vi "Main.vi"(11 "Module Admin":refnum<class "Delacor_lib_QMH_Cloneable Module Admin.lvclass">) -> ()   [LabVIEW 2024, in "OtroClon.lvlib"]
doc: "This template is based off of the Queued Message Handler design pattern and the Queued Message Handler project template that ships with LabVIEW.\n\nThe main difference is that the queue is private to this module and communication between modules is performed via Broadcast and Request events.\n\nRequest events are wrapped in public API methods and are handled in the Event Handling Loop (EHL) of this VI. Any module can register for Broadcast events sent by this module. The EHL generates messages based on user interface actions.\n\nThe Message Handling Loop (MHL) processes messages generated by the EHL, or by other messages. The messages are string values, so new messages can be added easily to the Message Cases case structure in the MHL. Each message cluster can also provide an optional value for Message Data, which is a variant that can be converted to whatever message-specific data is required.\n_____\nBased on DQMH Dev Tools: Project Template 7.1.0.1503."
uses:
  OtroClon.lvlib
  <vilib>/Delacor/Delacor QMH/Libraries/Cloneable Module Admin_class/Delacor_lib_QMH_Cloneable Module Admin.lvclass
  C:/Program Files (x86)/National Instruments/LabVIEW 2024/vi.lib/Delacor/Delacor QMH/Libraries/Module Admin_class/Delacor_lib_QMH_Module Admin.lvclass
  Module Data--cluster.ctl
  Do Something Argument--cluster.ctl
  <vilib>/Delacor/Delacor QMH/Libraries/Cloneable Module Admin_class/Delacor_lib_QMH_Cloneable Module Admin.lvclass/Delacor_lib_QMH_Cloneable Module Admin.ctl
  <vilib>/Delacor/Delacor QMH/Libraries/Message Queue_class/Delacor_lib_QMH_Message Queue.lvclass/Delacor_lib_QMH_Message Queue.ctl
  Do Something Else Argument--cluster.ctl
  Do Something Else and Wait for Reply Argument--cluster.ctl
  Do Something Else and Wait (Reply Payload)--cluster.ctl
  Stop Argument--cluster.ctl
  <vilib>/Delacor/Delacor QMH/Libraries/Module Admin_class/Delacor_lib_QMH_Module Admin.lvclass/Delacor_lib_QMH_Module Admin.ctl
  Evento Demo Copia Argument--cluster.ctl
  Set Signal Type Argument--cluster.ctl
  <vilib>/Utility/miscctls.llb/LVPointTypeDef.ctl
  <vilib>/Delacor/Delacor QMH/Libraries/Message Queue_class/Delacor_lib_QMH_Enqueue Message (Single).vi
  <vilib>/Delacor/Delacor QMH/Libraries/Cloneable Module Admin_class/Delacor_lib_QMH_Get Module ID.vi
  <vilib>/Delacor/Delacor QMH/Libraries/Module Admin_class/Delacor_lib_QMH_Get External Launch.vi
  <vilib>/Delacor/Delacor QMH/Libraries/Message Queue_class/Delacor_lib_QMH_Message Queue.lvclass
panel:
  out "error out":errorcluster
  out "X":dbl
  out "Status":string
  in  "Simulate EHL Error":bool
  in  "Simulate MHL Error":bool
  in  "Do Something Else <Replace Me>":bool
  in  "Do Something <Replace Me>":bool
  # "These controls have associated \"Value Changed\" events configured in the Event Structure on the diagram.\n\nReplace them (and reconfigure the Event Structure) with the controls you need for your application. \n\nOther processes communicate with this Module via its Public API (wrappers for its Request Events).\n\nThis Module communicates with other processes via its Broadcast Events.\nAny process that wants to receive these messages can register for this module's Broadcast events."
  # "This template is for the DQMH framework. See the block diagram for more information on how to use this template."
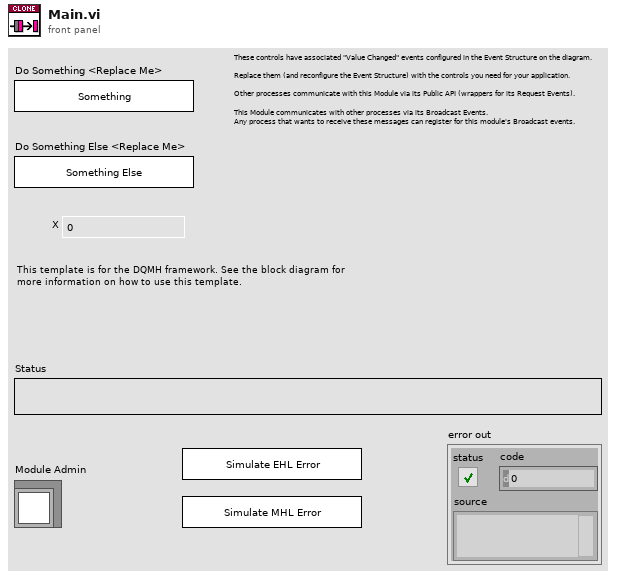
[diagram p1: front panel]
types:
  T1 = typedef "OtroClon.lvlib/Request Events--cluster.ctl" = cluster{"Stop Module":refnum<user-event>, "Do Something":refnum<user-event>, "Do Something Else":refnum<user-event>, "Do Something Else and Wait for Reply":refnum<user-event>, "Show Panel":refnum<user-event>, "Hide Panel":refnum<user-event>, "Show Diagram":refnum<user-event>, "Get Module Execution Status":refnum<user-event>, "Evento Demo Copia":refnum<user-event>, "Set Signal Type":refnum<user-event>}
  T2 = typedef "OtroClon.lvlib/Module Data--cluster.ctl" = cluster{"Status":string, "signal type":enum16{"Sine Wave", "Triangle Wave", "Square Wave", "Sawtooth Wave"}}
  T3 = typedef "OtroClon.lvlib/Do Something Argument--cluster.ctl" = cluster{"Module ID":i32, "Do Something Msg":string}
  T4 = typedef "OtroClon.lvlib/Do Something Else Argument--cluster.ctl" = cluster{"Module ID":i32, "Do Something Else Msg":string, "X":dbl}
  T5 = typedef "OtroClon.lvlib/Do Something Else and Wait for Reply Argument--cluster.ctl" = cluster{"Module ID":i32, "Do Something Else Msg":string, "X":dbl, "Wait Notifier":refnum<notifier>, "wait for reply":bool}
  T6 = enum32{"invalid lock state", "Not Locked", "Locked (No Password)", "Password-protected"}
  T7 = typedef "OtroClon.lvlib/Stop Argument--cluster.ctl" = cluster{"Module ID":i32, "Origin":string, "Exit via Stop Module Req?":bool, "Wait for Module to stop?":bool}
  T8 = typedef "OtroClon.lvlib/Evento Demo Copia Argument--cluster.ctl" = cluster{"Module ID":i32, "Numeric":dbl}
  T9 = typedef "OtroClon.lvlib/Set Signal Type Argument--cluster.ctl" = cluster{"Module ID":i32, "signal type":enum16{"Sine Wave", "Triangle Wave", "Square Wave", "Sawtooth Wave"}}
  T10 = typedef "LVPointTypeDef.ctl" = cluster{"Horizontal":i16, "Vertical":i16}
  T11 = enum32{"Invalid", "Standard", "Closed", "Hidden", "Minimized", "Maximized"}
  T12 = typedef "OtroClon.lvlib/Do Something Else and Wait (Reply Payload)--cluster.ctl" = cluster{"Value":dbl, "error":errorcluster, "Module ID":i32}
  T13 = enum16{"Sine Wave", "Triangle Wave", "Square Wave", "Sawtooth Wave"}
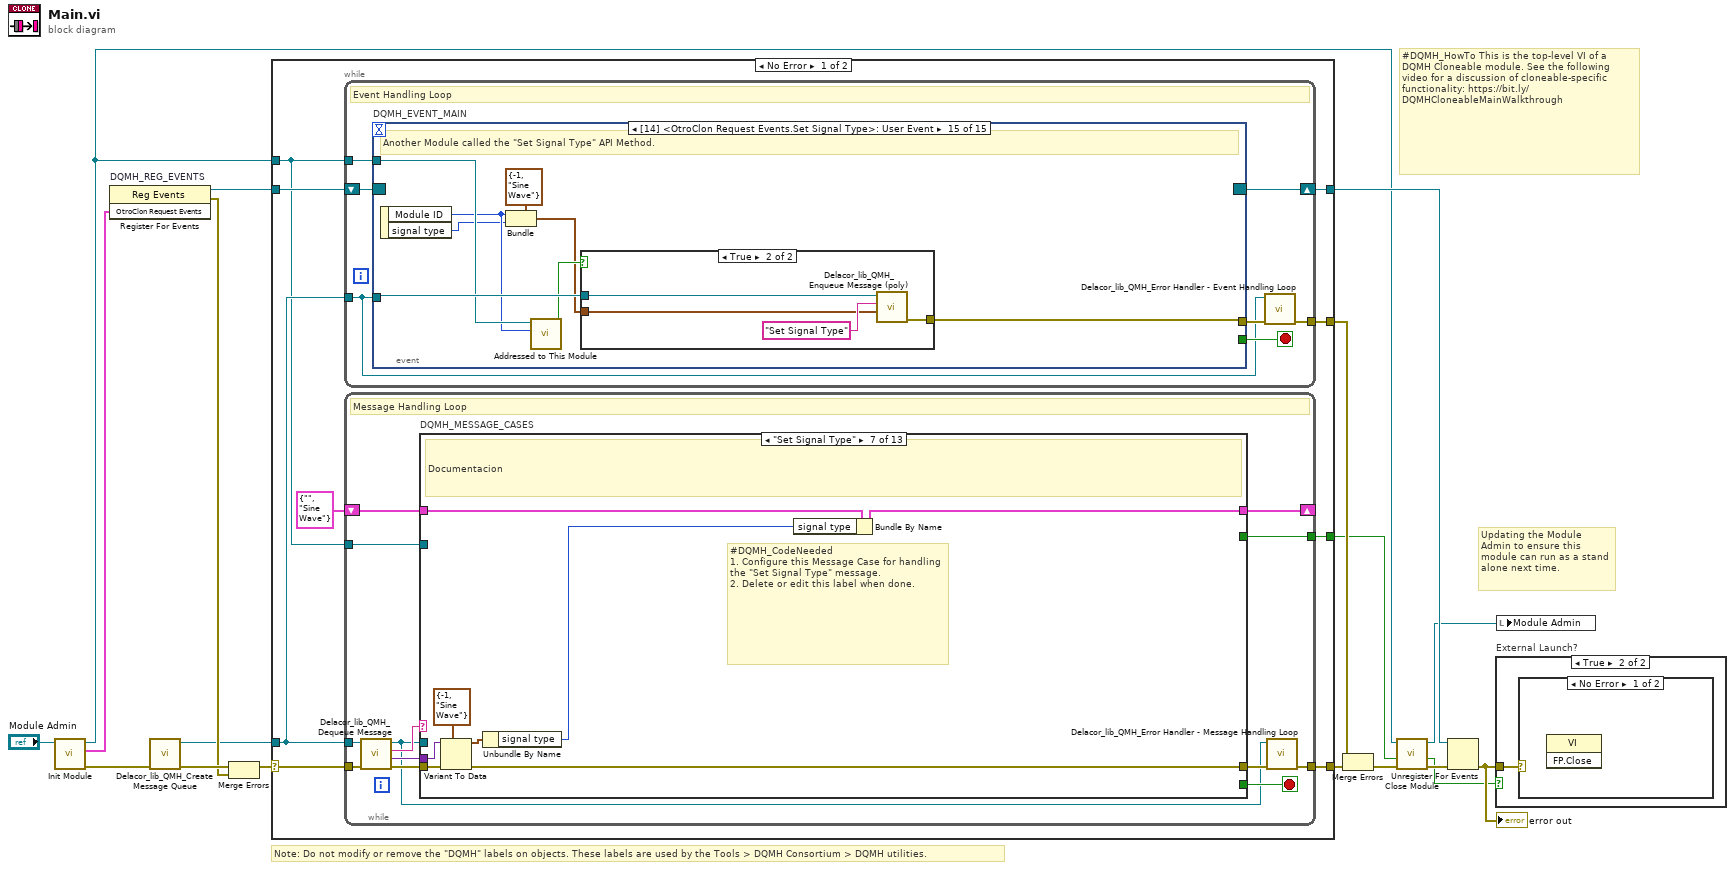
[diagram p0: block diagram]
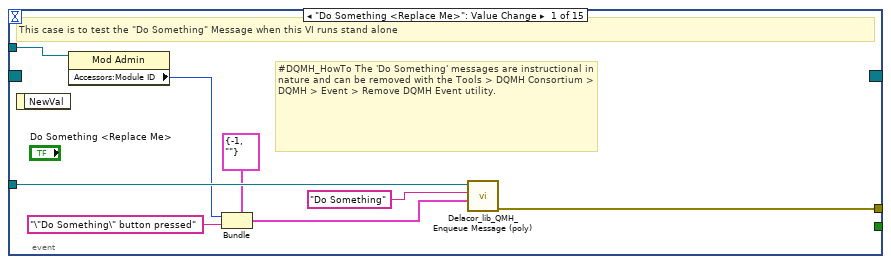
[diagram p2: hidden frame]
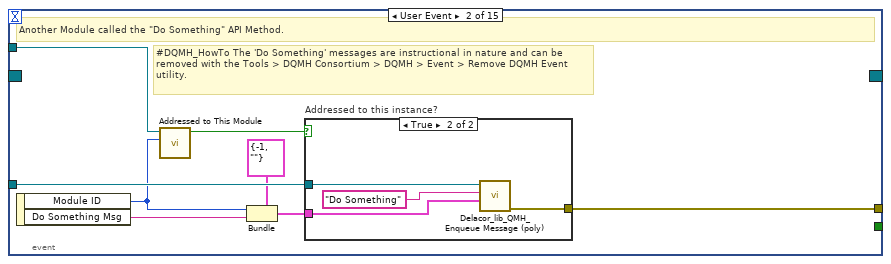
[diagram p3: hidden frame]
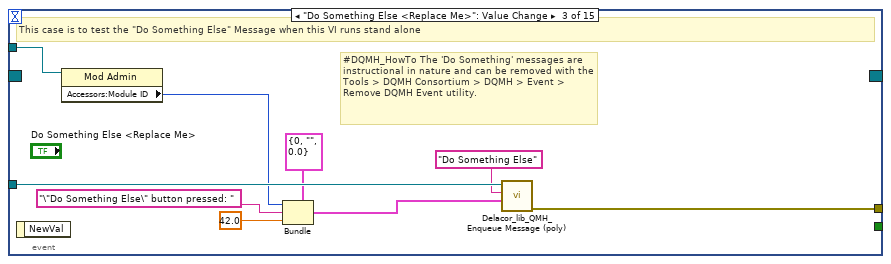
[diagram p5: hidden frame]
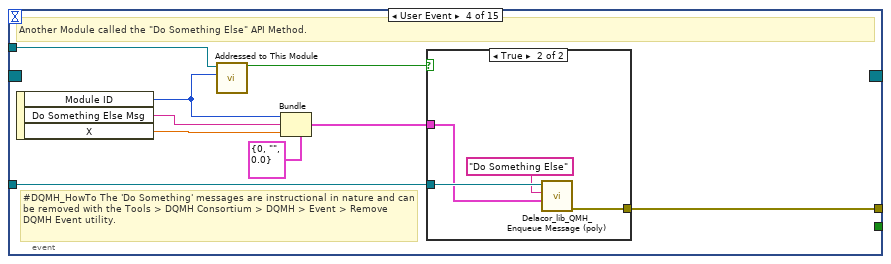
[diagram p6: hidden frame]
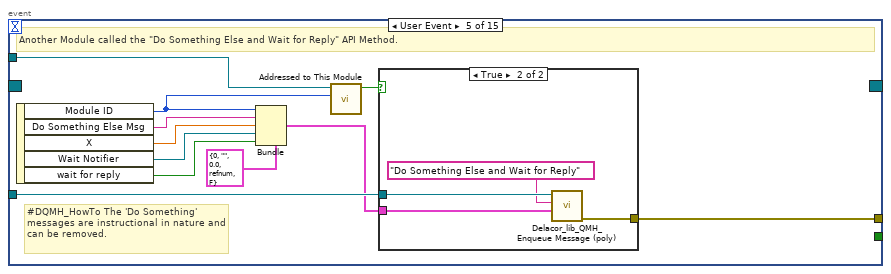
[diagram p8: hidden frame]
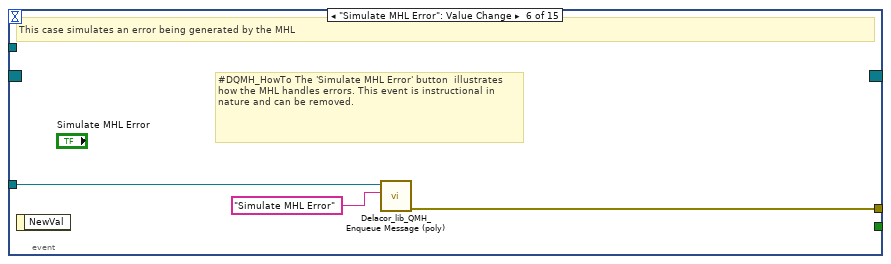
[diagram p10: hidden frame]
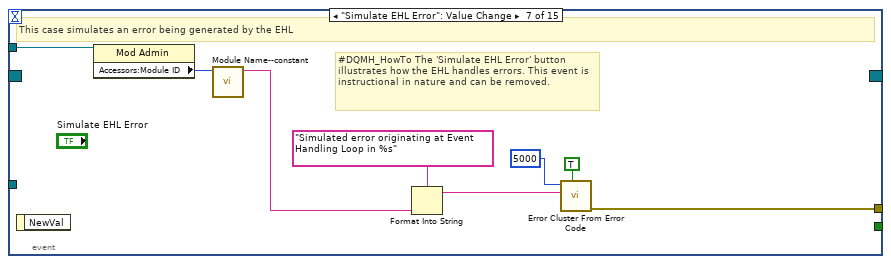
[diagram p11: hidden frame]
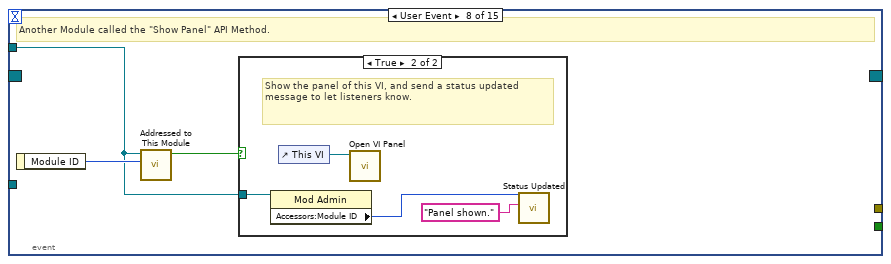
[diagram p12: hidden frame]
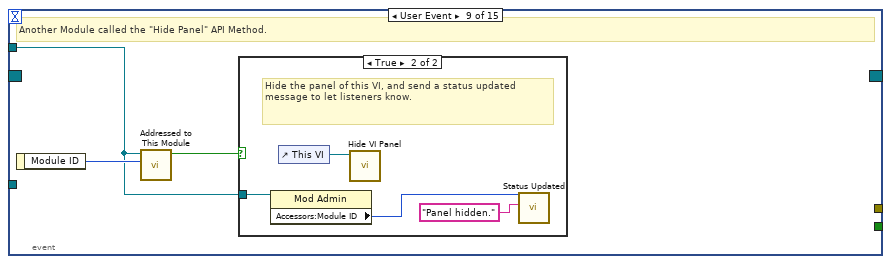
[diagram p14: hidden frame]
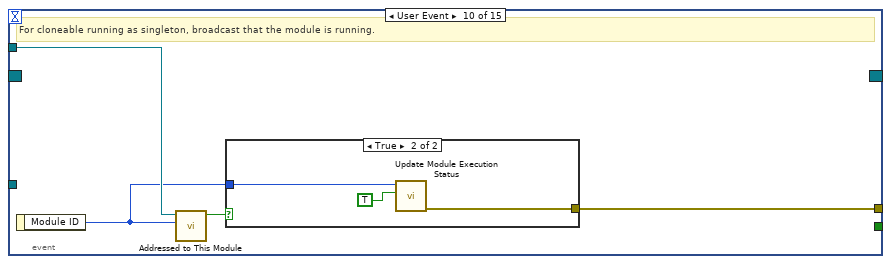
[diagram p16: hidden frame]
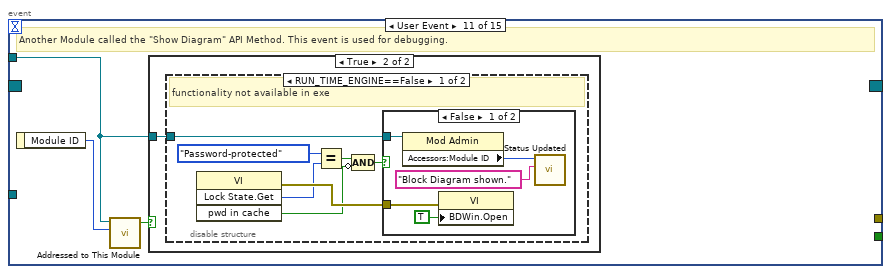
[diagram p18: hidden frame]
diagram:
  # "#DQMH_HowTo This is the top-level VI of a DQMH Cloneable module. See the following video for a discussion of cloneable-specific functionality: https://bit.ly/DQMHCloneableMainWalkthrough"
  # "Note: Do not modify or remove the \"DQMH\" labels on objects. These labels are used by the Tools > DQMH Consortium > DQMH utilities."
  # "Updating the Module Admin to ensure this module can run as a stand alone next time."
  n1 = call "Init Module.vi"("Cloneable Module Admin in"="Module Admin") -> ("error out"=w15:errorcluster, "OtroClon Request Events"=w7:T1, "Cloneable Module Admin out"=w4:refnum<class "Delacor_lib_QMH_Cloneable Module Admin.lvclass">)  [unwired: 8 in]
  n2 = register-events "DQMH_REG_EVENTS"(w7) -> (reference out=w8:refnum<event-registration>, error out=w10:errorcluster)  [unwired: 2 in]
  n3 = call <vilib>:"Delacor_lib_QMH_Create Message Queue.vi"("error in"=w15) -> ("error out"=w12:errorcluster, "Message Queue"=w6:refnum<class "Delacor_lib_QMH_Message Queue.lvclass">)  [unwired: 9 in]
  n4 = Merge Errors(w12, w10) -> (w11:errorcluster)
  n5 = case shown="No Error" w11 {
    selector: w11 -> [w25 w374]
    tunnel: [w27 w373] -> w16
    tunnel: [w24 w372] -> w9
    tunnel: w8 -> [w22 w372]
    tunnel: w6 -> [w21 w365]
    tunnel: [w26 _] -> w17
    tunnel: w4 -> [w20 w368]
    tunnel: [w19 _] -> w2
    frame No Error {
      n6 = while {
        tunnel: w21 -> [w28]
        shift-right: [w31] -> w24
        shift-left: w22 -> [w32]
        tunnel: [w33] -> w26
        tunnel: w20 -> [w29]
        stop <- w30 stop-if-true
        # "Event Handling Loop"
        n7 = event "DQMH_EVENT_MAIN" shown="[14] <OtroClon Request Events.Set Signal Type>: User Event" {
          selector: w32 -> [_ _ _ _ _ _ _ _ _ _ _ _ _ _ _]
          dyn-events: [_ _ _ _ _ _ _ _ _ _ _ _ _ _ _] -> w31
          timeout: _ -> [_ _ _ _ _ _ _ _ _ _ _ _ _ _ _]
          tunnel: [_ _ _ _ _ _ _ _ _ _ _ w143 _ _ _] -> w30
          tunnel: w28 -> [w41 w49 w62 w71 w86 w93 _ _ _ _ _ w146 w163 w183 w195]
          tunnel: [w42 w50 w63 w72 w87 w94 w102 _ _ w120 _ w147 w166 w176 w188] -> w34
          tunnel: w29 -> [w37 w47 w56 w69 w84 _ w101 w103 w110 w118 w124 w145 w164 w181 w193]
          event "Do Something <Replace Me>": Value Change {
            # "#DQMH_HowTo The 'Do Something' messages are instructional in nature and can be removed with the Tools > DQMH Consortium > DQMH > Event > Remove DQMH Event utility."
            # "This case is to test the \"Do Something\" Message when this VI runs stand alone"
            n8 = event-data() -> ()  [unwired: 1 in, 1 out]
            n9 = property on="Property Node" class="Mod Admin"(reference=w37) -> ("Accessors:Module ID"=w36:i32)  [unwired: 1 in, 2 out]
            n10 = Bundle(cluster=T3 {"Module ID"=-1, "Do Something Msg"=""} ("Do Something Argument"), "Module ID"=w36, "Do Something Msg"="\"Do Something\" button pressed" ("\"Do Something\" button pressed")) -> (w39:T3)
            n11 = call-poly <vilib>:"Delacor_lib_QMH_Enqueue Message (poly).vi"("Message Data"=w39, "Message"="Do Something", "Message Queue in"=w41) -> ("error out"=w42:errorcluster)  [unwired: 7 in, 1 out]
          }
          event User Event {
            # "#DQMH_HowTo The 'Do Something' messages are instructional in nature and can be removed with the Tools > DQMH Consortium > DQMH > Event > Remove DQMH Event utility."
            # "Another Module called the \"Do Something\" API Method."
            n12 = event-data() -> ("Module ID"=w44:i32, "Do Something Msg"=w43:string)  [unwired: 1 in]
            n13 = call "Addressed to This Module.vi"("Module ID from Argument"=w44, "Module Admin"=w47) -> ("Addressed to this instance?"=w48:bool)  [unwired: 8 in, 1 out]
            n14 = Bundle(cluster=T3 {"Module ID"=-1, "Do Something Msg"=""} ("Do Something Argument"), "Module ID"=w44, "Do Something Msg"=w43) -> (w46:T3)
            n15 = case "Addressed to this instance?" shown="True" w48 {
              tunnel: w49 -> [_ w53]
              tunnel: [_ w54] -> w50
              tunnel: w46 -> [_ w51]
              frame False {
                # "Do nothing"
              }
              frame True {
                n16 = call-poly <vilib>:"Delacor_lib_QMH_Enqueue Message (poly).vi"("Message Data"=w51, "Message"="Do Something", "Message Queue in"=w53) -> ("error out"=w54:errorcluster)  [unwired: 7 in, 1 out]
              }
            }
          }
          event "Do Something Else <Replace Me>": Value Change {
            # "#DQMH_HowTo The 'Do Something' messages are instructional in nature and can be removed with the Tools > DQMH Consortium > DQMH > Event > Remove DQMH Event utility."
            # "This case is to test the \"Do Something Else\" Message when this VI runs stand alone"
            n17 = event-data() -> ()  [unwired: 1 in, 1 out]
            n18 = property on="Property Node" class="Mod Admin"(reference=w56) -> ("Accessors:Module ID"=w55:i32)  [unwired: 1 in, 2 out]
            n19 = Bundle(cluster=T4 {"Module ID"=0, "Do Something Else Msg"="", "X"=0.0} ("Do Something Else Argument"), "Module ID"=w55, "Do Something Else Msg"="\"Do Something Else\" button pressed: " ("\"Do Something Else\" button pressed"), "X"=42.0) -> (w59:T4)
            n20 = call-poly <vilib>:"Delacor_lib_QMH_Enqueue Message (poly).vi"("Message Data"=w59, "Message"="Do Something Else", "Message Queue in"=w62) -> ("error out"=w63:errorcluster)  [unwired: 7 in, 1 out]
          }
          event User Event {
            # "#DQMH_HowTo The 'Do Something' messages are instructional in nature and can be removed with the Tools > DQMH Consortium > DQMH > Event > Remove DQMH Event utility."
            # "Another Module called the \"Do Something Else\" API Method."
            n21 = event-data() -> ("Module ID"=w64:i32, "Do Something Else Msg"=w65:string, "X"=w67:dbl)  [unwired: 1 in]
            n22 = call "Addressed to This Module.vi"("Module ID from Argument"=w64, "Module Admin"=w69) -> ("Addressed to this instance?"=w70:bool)  [unwired: 8 in, 1 out]
            n23 = Bundle(cluster=T4 {"Module ID"=0, "Do Something Else Msg"="", "X"=0.0} ("Do Something Else Argument"), "Module ID"=w64, "Do Something Else Msg"=w65, "X"=w67) -> (w66:T4)
            n24 = case shown="True" w70 {
              tunnel: w71 -> [_ w75]
              tunnel: [_ w76] -> w72
              tunnel: w66 -> [_ w73]
              frame False {
              }
              frame True {
                n25 = call-poly <vilib>:"Delacor_lib_QMH_Enqueue Message (poly).vi"("Message Data"=w73, "Message"="Do Something Else", "Message Queue in"=w75) -> ("error out"=w76:errorcluster)  [unwired: 7 in, 1 out]
              }
            }
          }
          event User Event {
            # "#DQMH_HowTo The 'Do Something' messages are instructional in nature and can be removed."
            # "Another Module called the \"Do Something Else and Wait for Reply\" API Method."
            n26 = event-data() -> ("Module ID"=w82:i32, "Do Something Else Msg"=w80:string, "X"=w79:dbl, "Wait Notifier"=w78:refnum<notifier>, "wait for reply"=w77:bool)  [unwired: 1 in]
            n27 = Bundle(cluster=T5 {"Module ID"=0, "Do Something Else Msg"="", "X"=0.0, "Wait Notifier"=refnum, "wait for reply"=FALSE} ("Do Something Else and Wait for Reply Argument"), "Module ID"=w82, "Do Something Else Msg"=w80, "X"=w79, "Wait Notifier"=w78, "wait for reply"=w77) -> (w81:T5)
            n28 = call "Addressed to This Module.vi"("Module ID from Argument"=w82, "Module Admin"=w84) -> ("Addressed to this instance?"=w85:bool)  [unwired: 8 in, 1 out]
            n29 = case shown="True" w85 {
              tunnel: [_ w91] -> w87
              tunnel: w86 -> [_ w90]
              tunnel: w81 -> [_ w88]
              frame False {
              }
              frame True {
                n30 = call-poly <vilib>:"Delacor_lib_QMH_Enqueue Message (poly).vi"("Message Data"=w88, "Message"="Do Something Else and Wait for Reply", "Message Queue in"=w90) -> ("error out"=w91:errorcluster)  [unwired: 7 in, 1 out]
              }
            }
          }
          event "Simulate MHL Error": Value Change {
            # "#DQMH_HowTo The 'Simulate MHL Error' button  illustrates how the MHL handles errors. This event is instructional in nature and can be removed."
            # "This case simulates an error being generated by the MHL"
            n31 = event-data() -> ()  [unwired: 1 in, 1 out]
            n32 = call-poly <vilib>:"Delacor_lib_QMH_Enqueue Message (poly).vi"("Message"="Simulate MHL Error", "Message Queue in"=w93) -> ("error out"=w94:errorcluster)  [unwired: 8 in, 1 out]
          }
          event "Simulate EHL Error": Value Change {
            # "#DQMH_HowTo The 'Simulate EHL Error' button  illustrates how the EHL handles errors. This event is instructional in nature and can be removed."
            # "This case simulates an error being generated by the EHL"
            n33 = event-data() -> ()  [unwired: 1 in, 1 out]
            n34 = property on="Property Node" class="Mod Admin"(reference=w101) -> ("Accessors:Module ID"=w100:i32)  [unwired: 1 in, 2 out]
            n35 = call "Module Name--constant.vi"("Module ID"=w100) -> ("Module Name"=w95:string)  [unwired: 10 in]
            n36 = Format Into String(format string="Simulated error originating at Event Handling Loop in %s", w95) -> (resulting string=w98:string)  [unwired: 2 in, 1 out]
            n37 = call <vilib>:"Error Cluster From Error Code.vi"("show call chain? (False)"=TRUE, "error message (\"\")"=w98, "error code (0)"=5000) -> ("error out"=w102:errorcluster)  [unwired: 6 in]
          }
          event User Event {
            # "Another Module called the \"Show Panel\" API Method."
            n38 = event-data() -> ("Module ID"=w104:i32)  [unwired: 1 in]
            n39 = call "Addressed to This Module.vi"("Module ID from Argument"=w104, "Module Admin"=w103) -> ("Addressed to this instance?"=w105:bool)  [unwired: 8 in, 1 out]
            n40 = case shown="True" w105 {
              tunnel: w103 -> [_ w107]
              frame False {
              }
              frame True {
                # "Show the panel of this VI, and send a status updated message to let listeners know."
                n41 = property on="Property Node" class="Mod Admin"(reference=w107) -> ("Accessors:Module ID"=w106:i32)  [unwired: 1 in, 2 out]
                n42 = control-ref of="This VI"() -> (w109:refnum<vi>)
                n43 = call "Open VI Panel.vi"("VI"=w109) -> ()  [unwired: 10 in, 1 out]
                n44 = call "Status Updated.vi"("Status"="Panel shown." ("format string"), "Module ID"=w106) -> ()  [unwired: 9 in, 1 out]
              }
            }
          }
          event User Event {
            # "Another Module called the \"Hide Panel\" API Method."
            n45 = event-data() -> ("Module ID"=w111:i32)  [unwired: 1 in]
            n46 = call "Addressed to This Module.vi"("Module ID from Argument"=w111, "Module Admin"=w110) -> ("Addressed to this instance?"=w112:bool)  [unwired: 8 in, 1 out]
            n47 = case shown="True" w112 {
              tunnel: w110 -> [_ w114]
              frame False {
              }
              frame True {
                # "Hide the panel of this VI, and send a status updated message to let listeners know."
                n48 = property on="Property Node" class="Mod Admin"(reference=w114) -> ("Accessors:Module ID"=w113:i32)  [unwired: 1 in, 2 out]
                n49 = control-ref of="This VI"() -> (w116:refnum<vi>)
                n50 = call "Hide VI Panel.vi"("VI"=w116) -> ()  [unwired: 10 in, 1 out]
                n51 = call "Status Updated.vi"("Status"="Panel hidden." ("format string"), "Module ID"=w113) -> ()  [unwired: 9 in, 1 out]
              }
            }
          }
          event User Event {
            # "For cloneable running as singleton, broadcast that the module is running."
            n52 = event-data() -> ("Module ID"=w117:i32)  [unwired: 1 in]
            n53 = call "Addressed to This Module.vi"("Module ID from Argument"=w117, "Module Admin"=w118) -> ("Addressed to this instance?"=w119:bool)  [unwired: 8 in, 1 out]
            n54 = case shown="True" w119 {
              tunnel: [_ w123] -> w120
              tunnel: w117 -> [_ w122]
              frame False {
              }
              frame True {
                n55 = call "Update Module Execution Status.vi"("Running?"=TRUE, "Module ID"=w122) -> ("error out"=w123:errorcluster)  [unwired: 9 in]
              }
            }
          }
          event User Event {
            # "Another Module called the \"Show Diagram\" API Method. This event is used for debugging."
            n56 = event-data() -> ("Module ID"=w125:i32)  [unwired: 1 in]
            n57 = call "Addressed to This Module.vi"("Module ID from Argument"=w125, "Module Admin"=w124) -> ("Addressed to this instance?"=w126:bool)  [unwired: 8 in, 1 out]
            n58 = case shown="True" w126 {
              tunnel: w124 -> [_ w127]
              frame False {
              }
              frame True {
                n59 = disable-structure shown="RUN_TIME_ENGINE==False" {
                  disable-tunnel: w127 -> [w128 _]
                  frame condition #0 (active) {
                    # "functionality not available in exe"
                    n60 = invoke on="Invoke Node" class="VI" method="Lock State.Get"() -> (error out=w134:errorcluster, "Get Lock State"=w133:T6, "pwd in cache"=w130:bool)  [unwired: 4 in, 1 out]
                    n61 = Equal?(x=T6."Password-protected", y=w133) -> (x = y?=w131:bool)
                    n62 = Compound Arithmetic op=AND(w131, invert w130) -> (w129:bool)
                    n63 = case shown="False" w129 {
                      tunnel: w134 -> [w139 _]
                      tunnel: w128 -> [w136 _]
                      frame False {
                        n64 = property on="Property Node" class="Mod Admin"(reference=w136) -> ("Accessors:Module ID"=w135:i32)  [unwired: 1 in, 2 out]
                        n65 = property on="Property Node" class="VI"(error in=w139, "BDWin.Open"=TRUE ("Block Diagram Window:Open")) -> ()  [unwired: 1 in, 2 out]
                        n66 = call "Status Updated.vi"("Status"="Block Diagram shown." ("format string"), "Module ID"=w135) -> ()  [unwired: 9 in, 1 out]
                      }
                      frame True {
                        # "Password-protected VI, and the password is not in the cache. Do not show the diagram."
                      }
                    }
                  }
                  frame condition #1 {
                  }
                }
              }
            }
          }
          event User Event {
            # "Another Module called the \"Stop Module\" API Method  or the Message Handling Loop below."
            n67 = event-data() -> ("Module ID"=w141:i32, "Wait for Module to stop?"=w142:bool, "Origin"=w140:string)  [unwired: 1 in]
            n68 = call "Addressed to This Module.vi"("Module ID from Argument"=w141, "Module Admin"=w145) -> ("Addressed to this instance?"=w144:bool)  [unwired: 8 in, 1 out]
            n69 = case shown="True" w144 {
              tunnel: [_ w159] -> w147
              tunnel: w146 -> [_ w155]
              tunnel: [_ TRUE] -> w143
              tunnel: w142 -> [_ w150]
              tunnel: w141 -> [_ w152]
              tunnel: w140 -> [_ w148]
              frame False {
              }
              frame True {
                # "The event can get fired from the Exit message. The queue gets destroyed there. In this case, the Enqueue VI will return error 1. It is safe to ignore, because the module is already exiting."
                n70 = local write "Status"(w148) -> ()
                n71 = Bundle By Name(cluster=T7 {"Module ID"=-1, "Origin"="", "Exit via Stop Module Req?"=FALSE, "Wait for Module to stop?"=FALSE} ("Stop Argument"), "Module ID"=w152, "Exit via Stop Module Req?"=TRUE, "Wait for Module to stop?"=w150) -> (w149:T7)
                n72 = call-poly <vilib>:"Delacor_lib_QMH_Enqueue Message (poly).vi"("Priority Message? (F)"=TRUE, "Message Data"=w149, "Message"="Exit", "Message Queue in"=w155) -> ("error out"=w160:errorcluster)  [unwired: 6 in, 1 out]
                n73 = call <vilib>:"Clear Errors.vi"("error in (no error)"=w160, "specific error code to clear (0: all)"=1) -> ("error out"=w159:errorcluster)  [unwired: 4 in, 1 out]
              }
            }
          }
          event Panel Close? {
            w165 = TRUE  # Discard the event, the MHL is responsible for closing and stopping this VI.
            # "Hide the panel or send the 'Exit' message if the user clicks the 'X' on the module main VI panel."
            n74 = event-data() -> ()  [unwired: 1 in, 1 out]
            n75 = property on="Property Node" class="Mod Admin"(reference=w164) -> (reference out=w161:refnum<class "Delacor_lib_QMH_Cloneable Module Admin.lvclass">, "Accessors:External Launch"=w162:bool)  [unwired: 1 in, 1 out]
            n76 = case shown="True" w162 {
              tunnel: w163 -> [_ w174]
              tunnel: [_ w175] -> w166
              tunnel: w161 -> [w169 _]
              frame True {
                # "If externally launched, clicking the 'X' hides the panel, but doesn't close it."
                n77 = property on="Property Node" class="Mod Admin"(reference=w169) -> ("Accessors:Module ID"=w168:i32)  [unwired: 1 in, 2 out]
                n78 = call "Status Updated.vi"("Status"="Panel hidden." ("format string"), "Module ID"=w168) -> ("error out"=w167:errorcluster)  [unwired: 9 in]
                n79 = control-ref of="This VI"() -> (w171:refnum<vi>)
                n80 = call "Hide VI Panel.vi"("error in"=w167, "VI"=w171) -> ()  [unwired: 9 in, 1 out]
              }
              frame False {
                # "If run as a stand-alone VI, clicking the panel 'X' stops the VI."
                n81 = call-poly <vilib>:"Delacor_lib_QMH_Enqueue Message (poly).vi"("Priority Message? (F)"=TRUE, "Message"="Exit", "Message Queue in"=w174) -> ("error out"=w175:errorcluster)  [unwired: 7 in, 1 out]
              }
            }
            n82 = event-data ("Event Filter Node")("Discard?"=w165) -> ()  [unwired: 1 in, 1 out]
          }
          event User Event {
            # "Another Module called the \"Evento Demo Copia\" API Method."
            n83 = event-data() -> ("Module ID"=w178:i32, "Numeric"=w177:dbl)  [unwired: 1 in]
            n84 = Bundle(cluster=T8 {"Module ID"=-1, "Numeric"=0.0} ("Evento Demo Copia Argument"), "Module ID"=w178, "Numeric"=w177) -> (w179:T8)
            n85 = call "Addressed to This Module.vi"("Module ID from Argument"=w178, "Module Admin"=w181) -> ("Addressed to this instance?"=w182:bool)  [unwired: 8 in, 1 out]
            n86 = case shown="True" w182 {
              tunnel: w183 -> [_ w187]
              tunnel: w179 -> [_ w185]
              tunnel: [_ w184] -> w176
              frame False {
              }
              frame True {
                n87 = call-poly <vilib>:"Delacor_lib_QMH_Enqueue Message (poly).vi"("Message Data"=w185, "Message"="Evento Demo Copia", "Message Queue in"=w187) -> ("error out"=w184:errorcluster)  [unwired: 7 in, 1 out]
              }
            }
          }
          event User Event {
            # "Another Module called the \"Set Signal Type\" API Method."
            n88 = event-data() -> ("Module ID"=w190:i32, "signal type"=w189:T13)  [unwired: 1 in]
            n89 = Bundle(cluster=T9 {"Module ID"=-1, "signal type"=enum."Sine Wave"} ("Set Signal Type Argument"), "Module ID"=w190, "signal type"=w189) -> (w191:T9)
            n90 = call "Addressed to This Module.vi"("Module ID from Argument"=w190, "Module Admin"=w193) -> ("Addressed to this instance?"=w194:bool)  [unwired: 8 in, 1 out]
            n91 = case shown="True" w194 {
              tunnel: w195 -> [_ w199]
              tunnel: w191 -> [_ w197]
              tunnel: [_ w196] -> w188
              frame False {
              }
              frame True {
                n92 = call-poly <vilib>:"Delacor_lib_QMH_Enqueue Message (poly).vi"("Message Data"=w197, "Message"="Set Signal Type", "Message Queue in"=w199) -> ("error out"=w196:errorcluster)  [unwired: 7 in, 1 out]
              }
            }
          }
        }
        n93 = call-dynamic "Delacor_lib_QMH_Error Handler - Event Handling Loop.vi"("error in"=w34, "Message Queue in"=w28) -> ("dup error in"=w33:errorcluster)  [unwired: 8 in, 1 out]
      }
      n94 = while {
        tunnel: w21 -> [w200]
        shift-right: [w207] -> _
        shift-left: T2 {"Status"="", "signal type"=enum."Sine Wave"} ("Data Cluster") -> [w208]
        tunnel: w25 -> [w211]
        tunnel: [w209] -> w27
        tunnel: w20 -> [w202]
        tunnel: [w201] -> w19
        stop <- w206 stop-if-true
        # "Message Handling Loop"
        n95 = call-dynamic "Delacor_lib_QMH_Dequeue Message.vi"("error in"=w211, "Message Queue in"=w200) -> ("error out"=w210:errorcluster, "Message Data"=w204:variant, "Message"=w205:string, "Message Queue out"=w203:refnum<class "Delacor_lib_QMH_Message Queue.lvclass">)  [unwired: 6 in]
        n96 = case "DQMH_MESSAGE_CASES" shown="\"Set Signal Type\"" w205 {
          selector: w205 -> [_ _ _ _ _ _ _ _ _ _ _ _ w354]
          tunnel: w203 -> [_ _ _ _ _ _ _ _ _ w309 _ w346 _]
          tunnel: w210 -> [w231 w235 w245 w256 w277 w293 w301 w304 w306 w318 w335 w352 w363]
          tunnel: [w229 w235 w243 w255 w276 w291 w299 w303 w306 w314 w334 w347 w364] -> w212
          tunnel: w208 -> [w222 w234 w242 w254 w257 w292 w300 w302 w305 w313 w332 w345 w361]
          tunnel: [w221 w234 w242 w254 w257 w292 w295 w302 w305 w313 w332 w345 w361] -> w207
          tunnel: [_ _ _ _ _ _ _ _ _ _ _ w344 _] -> w206
          tunnel: w204 -> [_ _ w241 w251 w271 w290 w298 _ _ w312 _ w342 _]
          tunnel: w202 -> [w217 _ w237 w247 w262 _ _ _ _ w311 w330 w337 w360]
          tunnel: [_ _ _ _ _ _ _ _ _ _ _ w340 _] -> w201
          frame "Initialize" {
            w214 = "Initial Message" ("Initial Message")
            # "#DQMH_CodeNeeded - Initialize the appearance of the front panel."
            # "#DQMH_CodeNeeded - Initialize your state data here."
            # "Initialize - Any operation that needs to be done before the module can receive messages. Synchronize Caller Events.vi will inform Start Module.vi that the module has launched and is ready to receive messages. Module Did Init.vi will broadcast that the module initialized."
            n97 = call "Synchronize Caller Events.vi"("error in"=w231, "Module Admin"=w217) -> ("error out"=w230:errorcluster, "Module Admin out"=w216:refnum<class "Delacor_lib_QMH_Cloneable Module Admin.lvclass">)  [unwired: 8 in]
            n98 = property on="Property Node" class="Mod Admin"(reference=w216) -> ("Accessors:Module ID"=w213:i32, "Accessors:External Launch"=w218:bool)  [unwired: 1 in, 2 out]
            n99 = call "Module Name--constant.vi"("Module ID"=w213) -> ("Module Name"=w226:string)  [unwired: 10 in]
            n100 = property on="Property Node" class="VI"("Front Panel.Title"=w226) -> (reference out=w228:refnum<vi>, error out=w233:errorcluster)  [unwired: 2 in]
            n101 = Select(t=T11."Hidden" ("State"), s=w218, f=T11."Standard" ("State")) -> (s? t:f=w223:T11)
            n102 = invoke on="Invoke Node" class="VI" method="FP.Open"(reference=w228, error in=w233, "State"=w223) -> (reference out=w227:refnum<vi>, error out=w232:errorcluster)  [unwired: 2 in, 3 out]
            n103 = Bundle By Name(cluster=w222, "Status"=w214) -> (w221:T2)
            n104 = invoke on="Invoke Node" class="VI" method="FP.Center"(reference=w227, error in=w232) -> ()  [unwired: 1 in, 3 out]
            n105 = property on="Pane" class="Pane"("Origin"=T10 {"Horizontal"=0, "Vertical"=0}) -> ()  [unwired: 2 in, 2 out]
            n106 = call "Module Name--constant.vi"("Module ID"=w213) -> ("Module Name"=w219:string)  [unwired: 10 in]
            n107 = call "Module Did Init.vi"("error in"=w230, "Initialized?"=TRUE, "Origin"=w219, "Module ID"=w213) -> ("error out"=w229:errorcluster)  [unwired: 7 in]
            "Status" <- w214
          }
          frame "---Module Specific---" {
            # "Separator -- The following cases handle messages specific to this Module."
          }
          frame "Do Something" {
            # "#DQMH_HowTo The 'Do Something' messages are instructional in nature and can be removed with the Tools > DQMH Consortium > DQMH > Event > Remove DQMH Event utility."
            # "Do Something - Replace this message with functionality for your own application. Note that this message also fires the \"Did Something\" broadcast event."
            n108 = Variant To Data(error in=w245, type=T3 {"Module ID"=-1, "Do Something Msg"=""} ("Do Something Argument"), Variant=w241) -> (data=w240:T3, error out=w244:errorcluster)
            n109 = property on="Property Node" class="Mod Admin"(reference=w237) -> ("Accessors:Module ID"=w236:i32)  [unwired: 1 in, 2 out]
            n110 = Unbundle By Name(w240) -> ("Do Something Msg"=w238:string)
            n111 = call "Status Updated.vi"("Status"=w238, "Module ID"=w236) -> ()  [unwired: 9 in, 1 out]
            n112 = local write "Status"(w238) -> ()
            n113 = call "Did Something.vi"("error in"=w244, "Did Something Msg"=w238, "Module ID"=w236) -> ("error out"=w243:errorcluster)  [unwired: 8 in]
          }
          frame "Do Something Else" {
            # "#DQMH_HowTo The 'Do Something' messages are instructional in nature and can be removed with the Tools > DQMH Consortium > DQMH > Event > Remove DQMH Event utility."
            # "Do Something Else - Replace this message with functionality for your own application."
            n114 = Variant To Data(error in=w256, type=T4 {"Module ID"=0, "Do Something Else Msg"="", "X"=0.0} ("Do Something Else Argument"), Variant=w251) -> (data=w252:T4, error out=w255:errorcluster)
            n115 = Unbundle By Name(w252) -> ("Do Something Else Msg"=w250:string, "X"=w249:dbl)
            "X" <- w249
            n116 = property on="Property Node" class="Mod Admin"(reference=w247) -> ("Accessors:Module ID"=w246:i32)  [unwired: 1 in, 2 out]
            n117 = Format Into String(initial string=w250, w249) -> (resulting string=w248:string)  [unwired: 2 in, 1 out]
            n118 = call "Status Updated.vi"("Status"=w248, "Module ID"=w246) -> ()  [unwired: 9 in, 1 out]
            n119 = local write "Status"(w248) -> ()
          }
          frame "Do Something Else and Wait for Reply" {
            w264 = "X(%.2f)+Offset(%.2f)=%.2f"  # status message format string
            # "#DQMH_HowTo The 'Do Something' messages are instructional in nature and can be removed."
            # "Send back X with a random offset"
            # "Do Something Else and Wait for Reply - Replace this message with functionality for your own application. Note that this message must fire a notifier to let callers know it has finished execution, and it returns an error if the 'Value' is negative."
            n120 = property on="Property Node" class="Mod Admin"(reference=w262) -> ("Accessors:Module ID"=w259:i32)  [unwired: 1 in, 2 out]
            n121 = Variant To Data(error in=w277, type=T5 {"Module ID"=0, "Do Something Else Msg"="", "X"=0.0, "Wait Notifier"=refnum, "wait for reply"=FALSE} ("Do Something Else and Wait for Reply Argument"), Variant=w271) -> (data=w272:T5, error out=w275:errorcluster)
            n122 = Unbundle By Name(w272) -> ("Wait Notifier"=w269:refnum<notifier>, "Do Something Else Msg"=w270:string, "X"=w266:dbl, "wait for reply"=w260:bool)
            n123 = Random Number (0-1)() -> (number: 0 to 1=w265:dbl)
            n124 = Add(x=w265, y=w266) -> (x+y=w261:dbl)
            n125 = Less Than 0?(x=w261) -> (x < 0?=w258:bool)
            n126 = local write "X"(w266) -> ()
            n127 = case shown="True" w258 {
              tunnel: [_ w281] -> w274
              frame False {
              }
              frame True {
                n128 = call <vilib>:"Error Cluster From Error Code.vi"("show call chain? (False)"=TRUE, "error message (\"\")"="The 'Something Else and Wait for Reply' message generated a negative number, which is considered an error condition.", "error code (0)"=5000) -> ("error out"=w281:errorcluster)  [unwired: 6 in]
              }
            }
            n129 = Format Into String(format string=w264, initial string=w270, w266, w265, w261) -> (resulting string=w263:string)  [unwired: 1 in, 1 out]
            n130 = Bundle By Name(cluster=T12 {"Value"=0.0, "error"={"status"=FALSE, "code"=0, "source"=""}, "Module ID"=0} ("notification"), "error"=w274, "Value"=w261, "Module ID"=w259) -> (w267:T12)
            n131 = call "Status Updated.vi"("Status"=w263, "Module ID"=w259) -> ()  [unwired: 9 in, 1 out]
            n132 = local write "Status"(w263) -> ()
            n133 = case shown="True" w260 {
              tunnel: w269 -> [_ w285]
              tunnel: w267 -> [_ w284]
              frame False {
              }
              frame True {
                # "Simulate an operation that requires a wait."
                n134 = flat-sequence {
                  tunnel: w285 -> [w287]
                  tunnel: w284 -> [w286]
                  tunnel: w282 -> [_]
                  frame #0 {
                    n135 = Send Notification(notification=w286, notifier=w287) -> ()  [unwired: 1 in, 2 out]
                  }
                }
                n136 = Wait (ms)(milliseconds to wait=u32 1000) -> (millisecond timer value=w282:u32)
              }
            }
            n137 = Merge Errors(w275, w274) -> (w276:errorcluster)
          }
          frame "Evento Demo Copia" {
            # "#DQMH_CodeNeeded\n1. Configure this Message Case for handling the \"Evento Demo Copia\" message.\n2. Delete or edit this label when done."
            # "este es una copia\n_____\nCreated using DQMH Framework: Event Scripter 7.1.0.1503."
            n138 = Variant To Data(error in=w293, type=T8 {"Module ID"=-1, "Numeric"=0.0} ("Evento Demo Copia Argument"), Variant=w290) -> (data=w288:T8, error out=w291:errorcluster)
            n139 = Unbundle By Name(w288) -> ()  [unwired: 2 out]
          }
          frame "Set Signal Type" {
            # "#DQMH_CodeNeeded\n1. Configure this Message Case for handling the \"Set Signal Type\" message.\n2. Delete or edit this label when done."
            # "Documentacion"
            n140 = Variant To Data(error in=w301, type=T9 {"Module ID"=-1, "signal type"=enum."Sine Wave"} ("Set Signal Type Argument"), Variant=w298) -> (data=w296:T9, error out=w299:errorcluster)
            n141 = Unbundle By Name(w296) -> ("signal type"=w294:T13)
            n142 = Bundle By Name(cluster=w300, "signal type"=w294) -> (w295:T2)
          }
          frame "---Copy This Frame---" {
            # "Duplicate this frame when creating new messages.  Change this comment in the duplicated frame to describe this message."
            n143 = Merge Errors(w304) -> (w303:errorcluster)
          }
          frame "---Exit and Error Handling---" {
            # "Separator - the following cases handle errors and exit messages."
          }
          frame "Error" {
            # "#DQMH_CodeRecommended - If the module is running in standalone mode (External Launch = FALSE), this code will pop up an error dialog and call the 'Exit' message if an error occurs. Add more fine-grained error management here."
            # "Error - Check the error message data and respond accordingly. This message is sent by the \"Error Handler\" VIs at the end of each loop in this application."
            n144 = property on="Property Node" class="Mod Admin"(reference=w311) -> ("Accessors:External Launch"=w310:bool, "Accessors:Module ID"=w308:i32)  [unwired: 1 in, 2 out]
            n145 = Variant To Data(error in=w318, type=errorcluster {"status"=FALSE, "code"=0, "source"=""} ("error constant"), Variant=w312) -> (data=w307:errorcluster, error out=w316:errorcluster)
            n146 = local write "error out"(w307) -> ()
            n147 = call "Error Reported.vi"("Error"=w307, "Module ID"=w308) -> ()  [unwired: 9 in, 1 out]
            n148 = case shown="False" w310 {
              tunnel: [w323 _] -> w315
              tunnel: w309 -> [w321 _]
              tunnel: w307 -> [w322 _]
              frame False {
                n149 = disable-structure shown="Default" {
                  disable-tunnel: w322 -> [w324 _]
                  frame condition #0 (active) {
                    # "If the module is running standalone, then pop up an error dialog and call the \"Exit\" message."
                    n150 = call <vilib>:"Simple Error Handler.vi"("error in (no error)"=w324) -> ()  [unwired: 4 in, 5 out]
                  }
                  frame condition #1 {
                    # "To prevent the Simple Error Handler VI from being loaded (e.g. when deploying to a Real-Time target), add the Conditional Disable Symbol \"DQMH_Disable_SEH\" to your project and set it to TRUE."
                  }
                }
                n151 = call-poly <vilib>:"Delacor_lib_QMH_Enqueue Message (poly).vi"("Priority Message? (F)"=TRUE, "Message"="Exit", "Message Queue in"=w321) -> ("error out"=w323:errorcluster)  [unwired: 7 in, 1 out]
              }
              frame True {
                # "If the module was launched externally, calling the Error Reported broadcast VI is the only action performed by the \"Error\" message. The module's caller can then process the error appropriately."
              }
            }
            n152 = Merge Errors(w316, w315) -> (w314:errorcluster)
          }
          frame "Simulate MHL Error" {
            # "#DQMH_HowTo The 'Simulate MHL Error' button  illustrates how the MHL handles errors. This event is instructional in nature and can be removed."
            # "Simulate an error occurring at the MHL"
            n153 = property on="Property Node" class="Mod Admin"(reference=w330) -> ("Accessors:Module ID"=w331:i32)  [unwired: 1 in, 2 out]
            n154 = call "Module Name--constant.vi"("Module ID"=w331) -> ("Module Name"=w326:string)  [unwired: 10 in]
            n155 = Format Into String(format string="Simulated error originating at Message Handling Loop in %s", w326) -> (resulting string=w327:string)  [unwired: 2 in, 1 out]
            n156 = call <vilib>:"Error Cluster From Error Code.vi"("show call chain? (False)"=TRUE, "error message (\"\")"=w327, "error code (0)"=5001) -> ("error out"=w333:errorcluster)  [unwired: 6 in]
            n157 = Merge Errors(w335, w333) -> (w334:errorcluster)
          }
          frame "Exit" {
            w343 = 91  # 91: not all Exit messages will have an argument
            w344 = TRUE  # Stop the VI
            # "Release the message queue reference"
            # "#DQMH_CodeNeeded - Add any required cleanup code here."
            # "Exit - Exit the application."
            n158 = Variant To Data(error in=w352, type=T7 {"Module ID"=-1, "Origin"="", "Exit via Stop Module Req?"=FALSE, "Wait for Module to stop?"=FALSE} ("Stop Argument"), Variant=w342) -> (data=w339:T7, error out=w348:errorcluster)
            n159 = call <vilib>:"Clear Errors.vi"("error in (no error)"=w348, "specific error code to clear (0: all)"=w343) -> ("error out"=w351:errorcluster)  [unwired: 4 in, 1 out]
            n160 = property on="Property Node" class="Mod Admin"(reference=w337) -> ("Accessors:Module ID"=w336:i32)  [unwired: 1 in, 2 out]
            n161 = control-ref of="This VI"() -> (w338:refnum<vi>)
            n162 = call-dynamic "Delacor_lib_QMH_Release Message Queue.vi"("error in"=w351, "Message Queue"=w346) -> ("error out"=w350:errorcluster)  [unwired: 9 in]
            n163 = call "Handle Exit.vi"("Stop Argument"=w339, "Module Admin in"=w337, "VI reference"=w338) -> ("error out"=w349:errorcluster, "Wait for Stop?"=w340:bool)  [unwired: 7 in]
            n164 = Merge Errors(w350, w349) -> (w347:errorcluster)
            n165 = call "Error Reported.vi"("Error"=w347, "Module ID"=w336) -> ()  [unwired: 9 in, 1 out]
          }
          frame Default {
            # "'Default' case only runs if there is a message that isn't defined in any of the other cases.  Output a programming error."
            n166 = property on="Property Node" class="Mod Admin"(reference=w360) -> ("Accessors:Module ID"=w359:i32)  [unwired: 1 in, 2 out]
            n167 = call "Module Name--constant.vi"("Module ID"=w359) -> ("Module Name"=w353:string)  [unwired: 10 in]
            n168 = Format Into String(format string="The invalid message string \"%s\" was received in the Message Handling Loop for module \"%s\".", w354, w353) -> (resulting string=w356:string)  [unwired: 2 in, 1 out]
            n169 = call <vilib>:"Error Cluster From Error Code.vi"("show call chain? (False)"=TRUE, "error message (\"\")"=w356, "error code (0)"=1) -> ("error out"=w362:errorcluster)  [unwired: 6 in]
            n170 = Merge Errors(w363, w362) -> (w364:errorcluster)
          }
        }
        n171 = call-dynamic "Delacor_lib_QMH_Error Handler - Message Handling Loop.vi"("error in"=w212, "Message Queue in"=w203) -> ("dup error in"=w209:errorcluster)  [unwired: 8 in, 1 out]
      }
    }
    frame Error {
      n172 = call "Synchronize Caller Events.vi"("Module Admin"=w368) -> ("Module Admin out"=w367:refnum<class "Delacor_lib_QMH_Cloneable Module Admin.lvclass">)  [unwired: 9 in, 1 out]
      n173 = property on="Property Node" class="Mod Admin"(reference=w367) -> ("Accessors:Module ID"=w366:i32)  [unwired: 1 in, 2 out]
      n174 = call-dynamic "Delacor_lib_QMH_Release Message Queue.vi"("error in"=w374, "Message Queue"=w365) -> ("error out"=w373:errorcluster)  [unwired: 9 in]
      n175 = call "Module Name--constant.vi"("Module ID"=w366) -> ("Module Name"=w371:string)  [unwired: 10 in]
      n176 = Format Into String(format string="An error occurred during initialization. %s is no longer running.", w371) -> (resulting string=w369:string)  [unwired: 2 in, 1 out]
      n177 = call "Error Reported.vi"("Additional Information"=w369, "Error"=w373, "Module ID"=w366) -> ()  [unwired: 8 in, 1 out]
    }
  }
  n178 = Merge Errors(w17, w16) -> (w18:errorcluster)
  n179 = call "Close Module.vi"("error in"=w18, "Wait for stop?"=w2, "Module Admin in"=w4) -> ("error out"=w14:errorcluster, "External Launch"=w1:bool, "Module Admin out"=w3:refnum<class "Delacor_lib_QMH_Cloneable Module Admin.lvclass">)  [unwired: 6 in]
  n180 = Unregister For Events(event registration refnum=w9, error in=w14) -> (error out=w13:errorcluster)
  "error out" <- w13
  n181 = case "External Launch?" shown="True" w1 {
    tunnel: w13 -> [_ w375]
    frame False {
    }
    frame True {
      n182 = case shown="No Error" w375 {
        frame No Error {
          n183 = invoke class="VI" method="FP.Close"() -> ()  [unwired: 3 in, 3 out]
        }
        frame Error {
          n184 = disable-structure shown="Default" {
            frame condition #0 (active) {
              n185 = invoke class="VI" method="FP.Open"("Activate"=TRUE ("Activate?")) -> ()  [unwired: 4 in, 5 out]
            }
            frame condition #1 {
              # "Don't show panel on error if running inside a built EXE."
            }
          }
        }
      }
    }
  }
  n186 = local write "Module Admin"(w3) -> ()
